vi "Tree.VI"   [LabVIEW 2013, in "PV ActiveLine.lvlib"]
uses:
  <instrlib>/PV ActiveLine/PV ActiveLine.lvlib
  <instrlib>/PV ActiveLine/Public/Configure/PV ActiveLine - SetDegas (TPG361).vi
  <instrlib>/PV ActiveLine/Public/Configure/PV ActiveLine - FilterTime (TPG361).vi
  <instrlib>/PV ActiveLine/Public/Configure/PV ActiveLine - OffsetDisplay (TPG361).vi
  <instrlib>/PV ActiveLine/Public/Configure/PV ActiveLine - FullScaleRange (TPG361).vi
  <instrlib>/PV ActiveLine/Public/Configure/PV ActiveLine - CalibrationFactor (TPG361).vi
  <instrlib>/PV ActiveLine/Public/Configure/PV ActiveLine - OffsetCorrection (TPG361).vi
  <instrlib>/PV ActiveLine/Public/Action-Status/PV ActiveLine - Sensor On-Off (TPG361).vi
  <instrlib>/PV ActiveLine/Public/Data/PV ActiveLine - Gas Type Correction (TPG361).vi
  <instrlib>/PV ActiveLine/Public/Action-Status/PV ActiveLine - Display Resolution (TPG362).vi
panel:
  # "SEE DIAGRAM FOR VI TREE"
  # "TPG 361\nTPG 362"
  # "Pfeiffer Vacuum GmbH\n Berlinerstrasse 43\n D-35614 Asslar\n\n Telefon +49-6441/802-0\n Telefax +49-6441/802-1202\n Internet: http://www.pfeiffer-vacuum.de"
  # "07.01.2001 FPF"
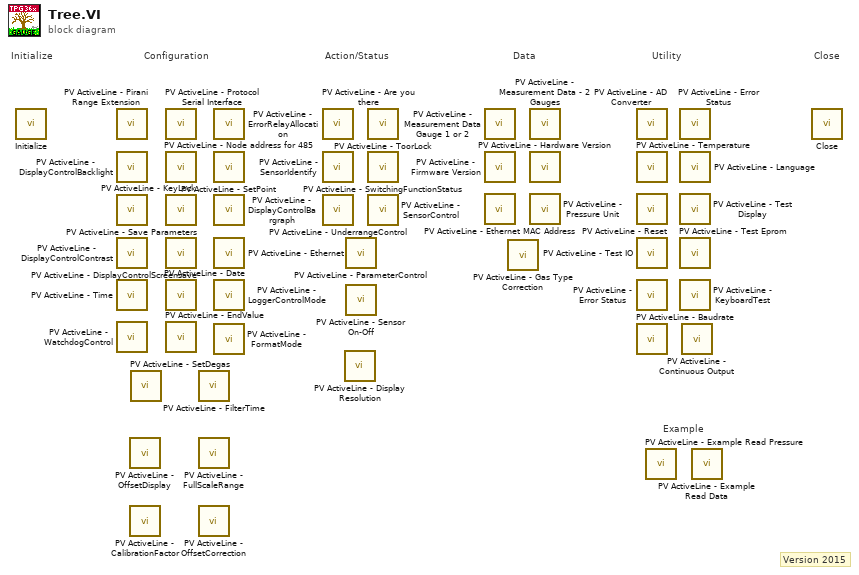
[diagram p0: block diagram]
diagram:
  # "Example"
  # "Configuration"
  # "Utility"
  # "Data"
  # "Action/Status"
  # "Close"
  # "Initialize"
  # "Version 2015"
  n1 = call <instrlib>:"Initialize.vi"() -> ()  [unwired: 10 in, 2 out]
  n2 = call <instrlib>:"PV ActiveLine - Pirani Range Extension.vi"() -> ()  [unwired: 9 in, 3 out]
  n3 = call <instrlib>:"PV ActiveLine - DisplayControlBacklight.vi"() -> ()  [unwired: 9 in, 3 out]
  n4 = call <instrlib>:"PV ActiveLine - Save Parameters.vi"() -> ()  [unwired: 8 in, 4 out]
  n5 = call <instrlib>:"PV ActiveLine - DisplayControlContrast.vi"() -> ()  [unwired: 9 in, 3 out]
  n6 = call <instrlib>:"PV ActiveLine - Time.vi"() -> ()  [unwired: 8 in, 4 out]
  n7 = call <instrlib>:"PV ActiveLine - WatchdogControl.vi"() -> ()  [unwired: 9 in, 3 out]
  n8 = call-poly <instrlib>:"PV ActiveLine - OffsetDisplay.vi"() -> ()  [unwired: 9 in, 3 out]
  n9 = call-poly <instrlib>:"PV ActiveLine - CalibrationFactor.vi"() -> ()  [unwired: 9 in, 3 out]
  n10 = call-poly <instrlib>:"PV ActiveLine - SetDegas.vi"() -> ()  [unwired: 9 in, 3 out]
  n11 = call <instrlib>:"PV ActiveLine - Protocol Serial Interface.vi"() -> ()  [unwired: 8 in, 4 out]
  n12 = call <instrlib>:"PV ActiveLine - Node address for 485.vi"() -> ()  [unwired: 8 in, 4 out]
  n13 = call <instrlib>:"PV ActiveLine - KeyLock.vi"() -> ()  [unwired: 8 in, 4 out]
  n14 = call <instrlib>:"PV ActiveLine - DisplayControlScreensave.vi"() -> ()  [unwired: 9 in, 3 out]
  n15 = call <instrlib>:"PV ActiveLine - Date.vi"() -> ()  [unwired: 11 in, 5 out]
  n16 = call <instrlib>:"PV ActiveLine - EndValue.vi"() -> ()  [unwired: 8 in, 4 out]
  n17 = call-poly <instrlib>:"PV ActiveLine - FilterTime.vi"() -> ()  [unwired: 9 in, 3 out]
  n18 = call-poly <instrlib>:"PV ActiveLine - FullScaleRange.vi"() -> ()  [unwired: 9 in, 3 out]
  n19 = call-poly <instrlib>:"PV ActiveLine - OffsetCorrection.vi"() -> ()  [unwired: 9 in, 3 out]
  n20 = call <instrlib>:"PV ActiveLine - ErrorRelayAllocation.vi"() -> ()  [unwired: 9 in, 3 out]
  n21 = call <instrlib>:"PV ActiveLine - SetPoint.vi"() -> ()  [unwired: 11 in, 5 out]
  n22 = call <instrlib>:"PV ActiveLine - DisplayControlBargraph.vi"() -> ()  [unwired: 9 in, 3 out]
  n23 = call <instrlib>:"PV ActiveLine - Ethernet.vi"() -> ()  [unwired: 10 in, 6 out]
  n24 = call <instrlib>:"PV ActiveLine - LoggerControlMode.vi"() -> ()  [unwired: 10 in, 6 out]
  n25 = call <instrlib>:"PV ActiveLine - FormatMode.vi"() -> ()  [unwired: 8 in, 4 out]
  n26 = call <instrlib>:"PV ActiveLine - Are you there.vi"() -> ()  [unwired: 9 in, 7 out]
  n27 = call <instrlib>:"PV ActiveLine - SensorIdentify.vi"() -> ()  [unwired: 8 in, 4 out]
  n28 = call <instrlib>:"PV ActiveLine - UnderrangeControl.vi"() -> ()  [unwired: 9 in, 3 out]
  n29 = call-poly <instrlib>:"PV ActiveLine - Display Resolution.vi"() -> ()  [unwired: 8 in, 4 out]
  n30 = call <instrlib>:"PV ActiveLine - ParameterControl.vi"() -> ()  [unwired: 9 in, 3 out]
  n31 = call-poly <instrlib>:"PV ActiveLine - Sensor On-Off.vi"() -> ()  [unwired: 9 in, 3 out]
  n32 = call <instrlib>:"PV ActiveLine - ToorLock.vi"() -> ()  [unwired: 9 in, 3 out]
  n33 = call <instrlib>:"PV ActiveLine - SwitchingFunctionStatus.vi"() -> ()  [unwired: 6 in, 6 out]
  n34 = call <instrlib>:"PV ActiveLine - SensorControl.vi"() -> ()  [unwired: 14 in, 6 out]
  n35 = call <instrlib>:"PV ActiveLine - Measurement Data Gauge 1 or 2.vi"() -> ()  [unwired: 8 in, 4 out]
  n36 = call <instrlib>:"PV ActiveLine - Firmware Version.vi"() -> ()  [unwired: 9 in, 3 out]
  n37 = call <instrlib>:"PV ActiveLine - Ethernet MAC Address.vi"() -> ()  [unwired: 3 in, 3 out]
  n38 = call-poly <instrlib>:"PV ActiveLine - Gas Type Correction.vi"() -> ()  [unwired: 9 in, 3 out]
  n39 = call <instrlib>:"PV ActiveLine - Measurement Data - 2 Gauges.vi"() -> ()  [unwired: 6 in, 6 out]
  n40 = call <instrlib>:"PV ActiveLine - Hardware Version.vi"() -> ()  [unwired: 9 in, 3 out]
  n41 = call <instrlib>:"PV ActiveLine - Pressure Unit.vi"() -> ()  [unwired: 9 in, 3 out]
  n42 = call <instrlib>:"PV ActiveLine - AD Converter.vi"() -> ()  [unwired: 8 in, 4 out]
  n43 = call <instrlib>:"PV ActiveLine - Temperature.vi"() -> ()  [unwired: 9 in, 3 out]
  n44 = call <instrlib>:"PV ActiveLine - Reset.vi"() -> ()  [unwired: 9 in, 3 out]
  n45 = call <instrlib>:"PV ActiveLine - Test IO.vi"() -> ()  [unwired: 8 in, 4 out]
  n46 = call <instrlib>:"PV ActiveLine - Error Status.vi"() -> ()  [unwired: 8 in, 4 out]
  n47 = call <instrlib>:"PV ActiveLine - Baudrate.vi"() -> ()  [unwired: 8 in, 4 out]
  n48 = call <instrlib>:"PV ActiveLine - Example Read Pressure.vi"() -> ()  [unwired: 9 in, 3 out]
  n49 = call <instrlib>:"PV ActiveLine - Error Status.vi"() -> ()  [unwired: 8 in, 4 out]
  n50 = call <instrlib>:"PV ActiveLine - Language.vi"() -> ()  [unwired: 8 in, 4 out]
  n51 = call <instrlib>:"PV ActiveLine - Test Display.vi"() -> ()  [unwired: 9 in, 3 out]
  n52 = call <instrlib>:"PV ActiveLine - Test Eprom.vi"() -> ()  [unwired: 8 in, 4 out]
  n53 = call <instrlib>:"PV ActiveLine - KeyboardTest.vi"() -> ()  [unwired: 6 in, 6 out]
  n54 = call <instrlib>:"PV ActiveLine - Continuous Output.vi"() -> ()  [unwired: 10 in, 2 out]
  n55 = call <instrlib>:"PV ActiveLine - Example Read Data.vi"() -> ()  [unwired: 9 in, 3 out]
  n56 = call <instrlib>:"Close.vi"() -> ()  [unwired: 11 in, 1 out]
